vi "st_eval CDF (poiss kx).vi"(4 "parameters":variant, 5 "x":dbl) -> (2 "f(x)":dbl)   [LabVIEW 2020, in "NI_Gmath.lvlib"]
uses:
  NI_Gmath.lvlib
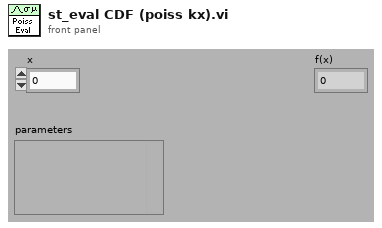
[diagram p1: front panel]
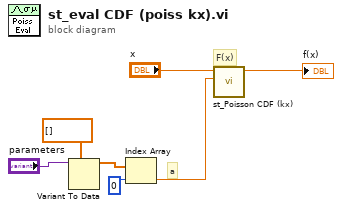
[diagram p0: block diagram]
diagram:
  # "a"
  # "F(x)"
  n1 = Variant To Data(type=dbl[] [], Variant="parameters") -> (data=w5:dbl[])  [unwired: 1 in, 1 out]
  n2 = Index Array(array=w5, index=0) -> (element=w1:dbl)
  n3 = call "st_Poisson CDF (kx).vi"("a"=w1, "x"="x") -> ("cdf(x)"=→"f(x)":dbl)  [unwired: 8 in, 1 out]
